vi "Get EventUniqueID.vi"(8 "error in (no error)":errorcluster, 11 "EventToken in":refnum<class "EventToken.lvclass">) -> (0 "error out":errorcluster, 2 "EventRefnum":i32, 3 "EventToken out":refnum<class "EventToken.lvclass">)   [LabVIEW 2021, in "EventManagerLibrary.lvlib" / "EventToken.lvclass"]
uses:
  EventToken.lvclass
  EventToken.lvclass/EventToken.ctl
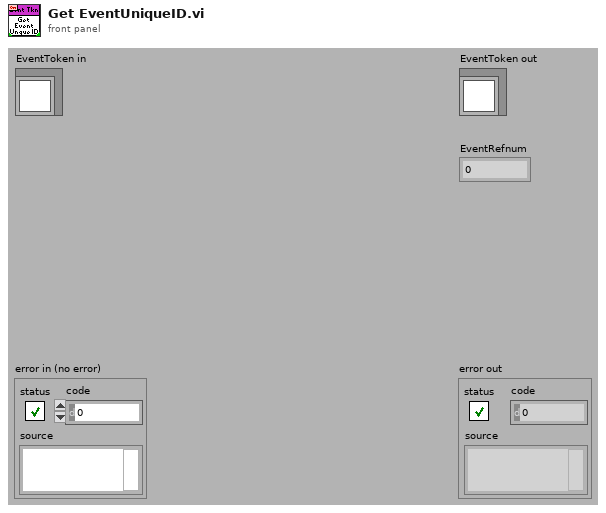
[diagram p1: front panel]
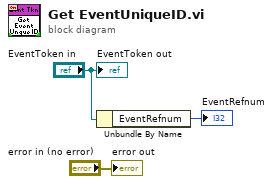
[diagram p0: block diagram]
diagram:
  n1 = Unbundle By Name("EventToken in") -> ("EventRefnum"=→"EventRefnum":i32)
  "error out" <- "error in (no error)"
  "EventToken out" <- "EventToken in"
